vi "基板箱读取条码.vi"(0 "开启条码?":bool=TRUE, 1 "VISA resource name":refnum<visa-resource-name>="COM1" caption="VISA资源名称") -> (7 "基板箱条码":string, 8 "基板箱NG？":bool)   [LabVIEW 2014]
uses:
  <vilib>/Instr/_visa.llb/VISA Configure Serial Port (Instr).vi
panel:
  out "错误输出":errorcluster
  out "读取缓冲区":string
  in  "termination char\n(0xA = '\\n' = LF)":u8=10 caption="终止符\n(0xA = '\\n' = LF)" format="%.0x"
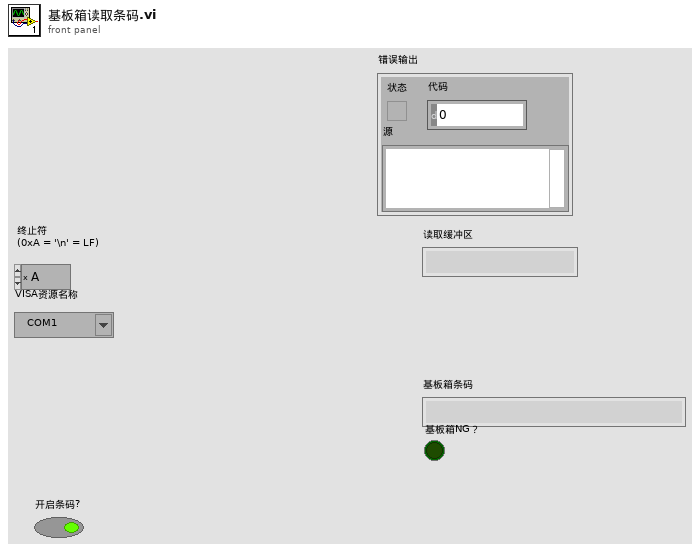
[diagram p1: front panel]
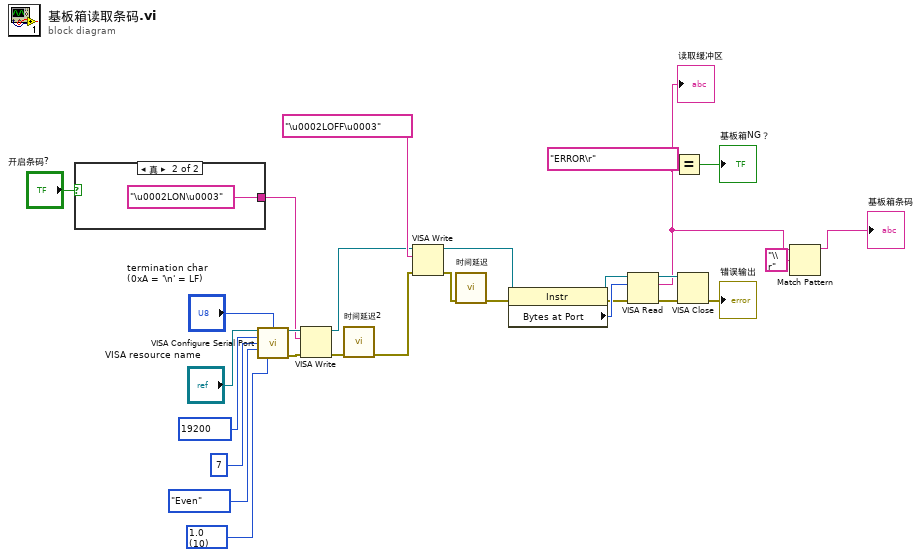
[diagram p0: block diagram]
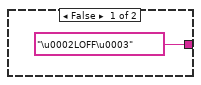
[diagram p2: hidden frame]
diagram:
  w23 = u16 10 items=["1.0"=10, "1.5"=15, "2.0"=20] ("stop bits (10: 1 bit)")
  n1 = case shown="真" "开启条码?" {
    tunnel: ["\u0002LOFF\u0003" "\u0002LON\u0003"] -> w19
    frame False {
    }
    frame True {
    }
  }
  n2 = call-poly "VISA Configure Serial Port"("VISA resource name"="VISA resource name", "termination char\n(0xA = '\\n' = LF)"="termination char\n(0xA = '\\n' = LF)", "baud rate (9600)"=u32 19200, "data bits (8)"=u16 7, "parity (0:none)"=enum16{"None", "Odd", "Even", "Mark", "Space"}."Even", "stop bits (10: 1 bit)"=w23) -> ("VISA resource name out"=w21:refnum<visa-resource-name>, "error out"=w20:errorcluster)  [unwired: 8 in]
  n3 = VISA Write(VISA resource name=w21, write buffer=w19, error in (no error)=w20) -> (VISA resource name out=w14:refnum<visa-resource-name>, error out=w18:errorcluster)  [unwired: 1 out]
  n4 = call "时间延迟2"("error in (no error)"=w18) -> ("error out"=w13:errorcluster)  [unwired: 10 in]
  n5 = VISA Write(VISA resource name=w14, write buffer="\u0002LOFF\u0003", error in (no error)=w13) -> (VISA resource name out=w8:refnum<visa-resource-name>, error out=w12:errorcluster)  [unwired: 1 out]
  n6 = call "时间延迟"("error in (no error)"=w12) -> ("error out"=w5:errorcluster)  [unwired: 10 in]
  n7 = property class="Instr"(reference=w8, error in=w5) -> (reference out=w6:refnum<visa-resource-name>, error out=w4:errorcluster, "Bytes at Port"=w7:u32)
  n8 = VISA Read(VISA resource name=w6, byte count=w7, error in (no error)=w4) -> (VISA resource name out=w11:refnum<visa-resource-name>, read buffer=w3:string, error out=w10:errorcluster)  [unwired: 1 out]
  "读取缓冲区" <- w3
  n9 = Equal?(x="ERROR\r", y=w3) -> (x = y?=→"基板箱NG？":bool)
  n10 = VISA Close(VISA resource name=w11, error in (no error)=w10) -> (error out=→"错误输出":errorcluster)
  n11 = Match Pattern(string=w3, regular expression="\\r" ("正则表达式")) -> (before substring=→"基板箱条码":string)  [unwired: 1 in, 3 out]
